vi "Third Flow Restarts Sandbox.vi"() -> ()   [LabVIEW 2013]
uses:
  Type Defs/CAN Mode.ctl
  Type Defs/Controller Names.ctl
  Type Defs/Controller List.ctl
  <vilib>/FPGAPlugInAG/sbRIO-9626/niLvFpga_Open_sbRIO-9626.vi
  <vilib>/rvi/interface/common/dynamic/niFpgaDynamicAddResources.vi
  <vilib>/rvi/interface/common/niFpgaWaitOnOcc.vi
  <vilib>/Utility/error.llb/Error Cluster From Error Code.vi
  <vilib>/rvi/errors/niLvFpgaAdjustHostInterfaceError.vi
  <vilib>/FPGAPlugInAG/Dynamic/niLvFpga_Reset_Dynamic.vi
  <vilib>/FPGAPlugInAG/Dynamic/niLvFpga_Run_Dynamic.vi
  <vilib>/rvi/interface/nirviOpenFPGA/nirviOpenFPGA.xnode
  FPGA/bitfiles/Third Flow Restart Sandbox.lvbitx
  <vilib>/rvi/interface/nirviMethod/nirviMethod.xnode
  <vilib>/rvi/interface/nirviReadWriteControl/nirviReadWriteControl.xnode
  NiFpgaLv.dll
  <vilib>/rvi/interface/Simulation/niFpgaSimulationCallBeginRW.vi
  <vilib>/NI_Real-Time Target Support.lvlib
  <vilib>/FPGAPlugInAG/Dynamic/niLvFpga_ReadFifo_Dynamic.vi
  <vilib>/rvi/errors/niLvFpgaMergeErrorWithErrorCode.vi
  <vilib>/FPGAPlugInAG/Dynamic/niLvFpga_ConfigureFifo_Dynamic.vi
panel:
  out "Cycles":i32
  in  "Reset Cycles":bool
  in  "Continue":bool
  out "Updating?":bool
  out "Starts":i32[](array[numeric])
  in  "Take Trace":bool
  out "tracker":u32
  out "Flow Graphs":dbl[][](graph)
  out "Current Graphs":dbl[][](graph)
  out "Restarts Graph":i32[][](graph)
  in  "Seconds per Step":dbl=1.5 min=0.25 max=500.0 step=0.25
  out "Case":string
  out "Current Step":i32
  in  "Reset Restarts":bool
  in  "Profile":dbl[][](array[numeric])=[[0.25, 0.0, 0.0, 1.0], [1.25, 650.0, 700.0, 0.0], [10.5, 0.0, 0.0, 0.0]]
  in  "Run profile?":bool
  out "CFR 2":u64 format="%.0x"
  in  "Pressure":dbl min=0.0 max=800.0 step=1.0 format="%#_13g"
  out "CPU Usage:":dbl=7.74131899555212 format="%.1f"
  in  "CAN CMD":dbl min=0.0 max=800.0 step=1.0
  # "cmd"
  # "pres"
  # "trigger"
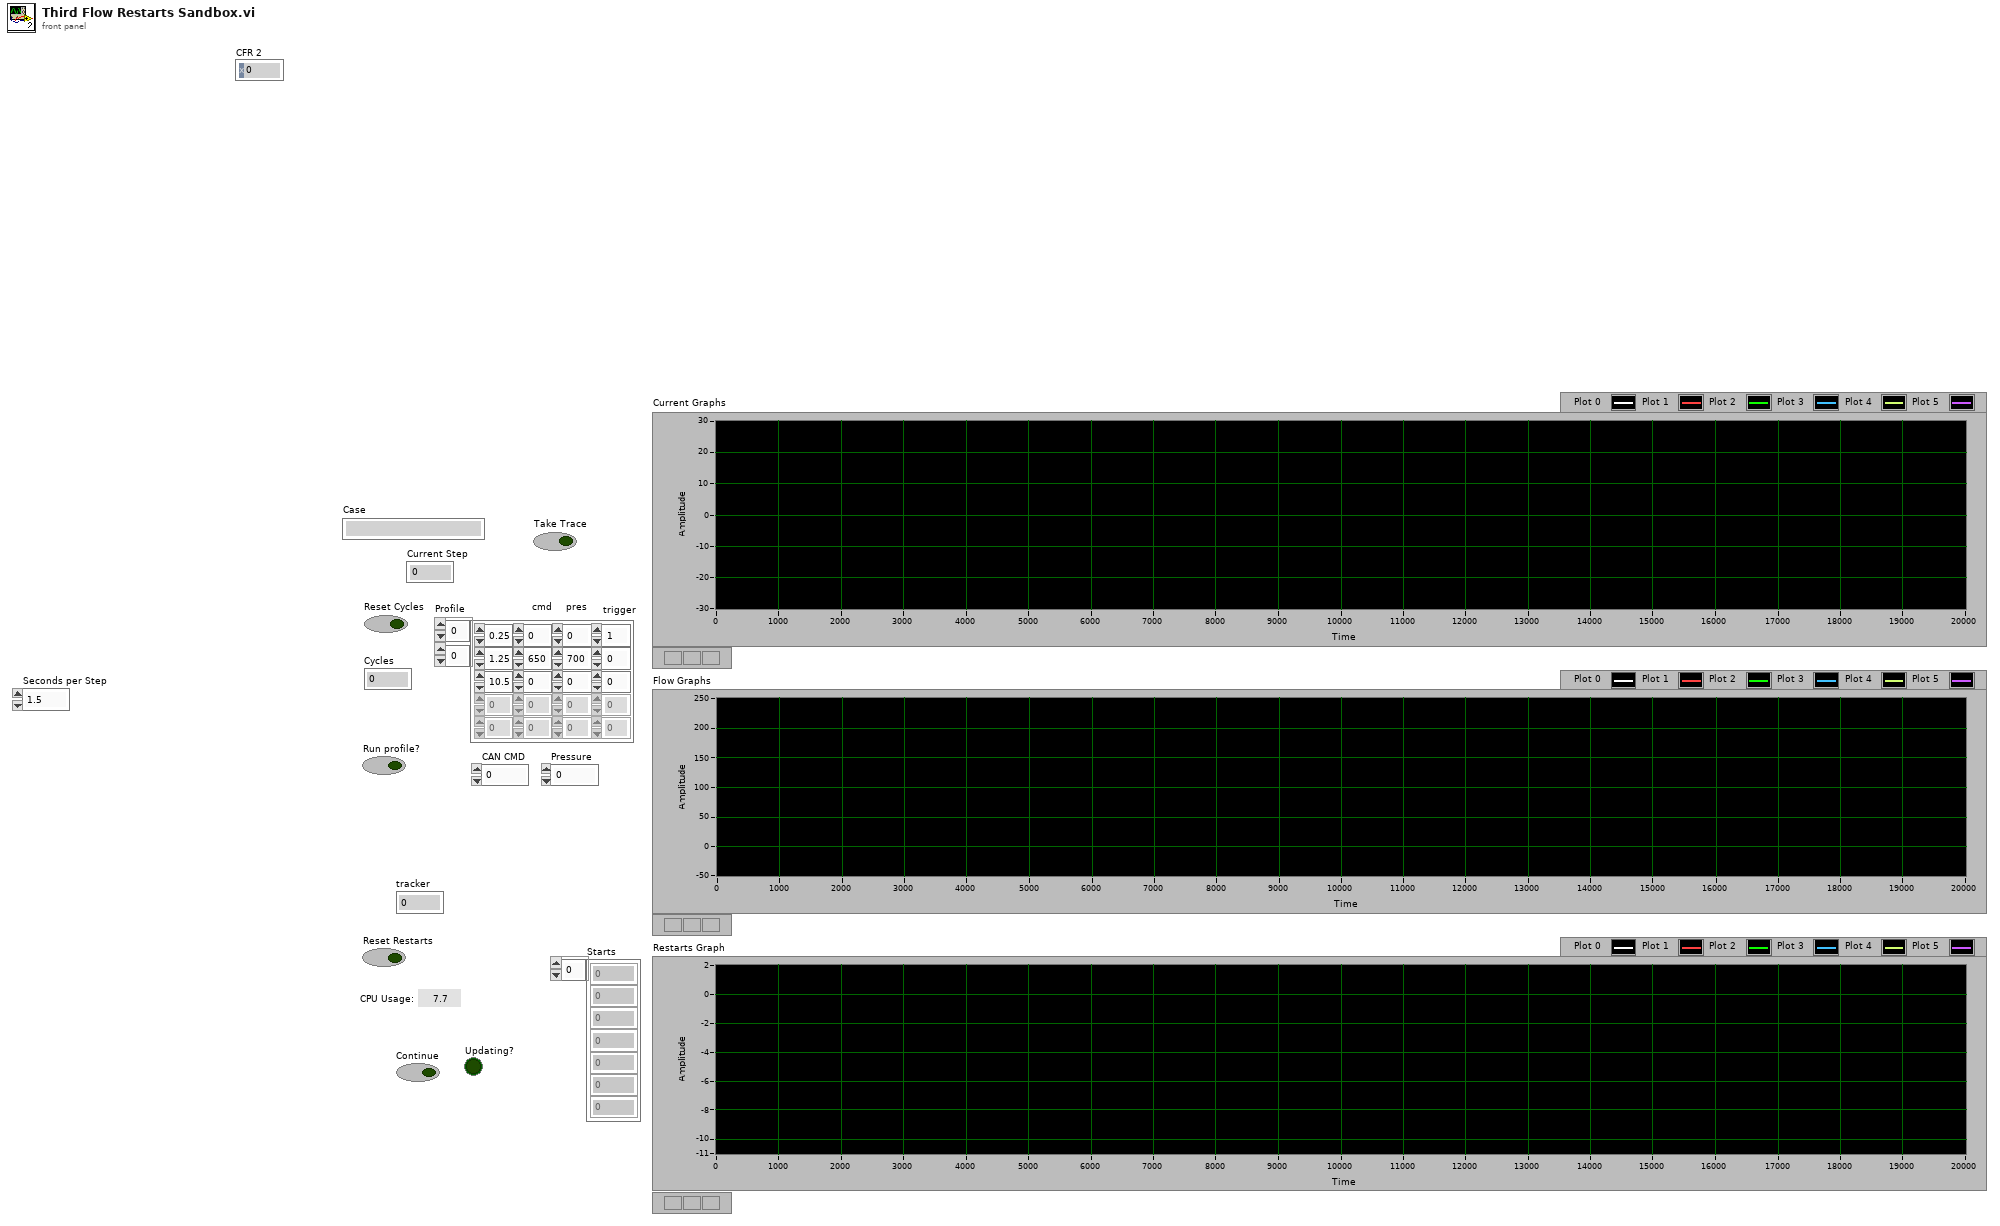
[diagram p1: front panel]
types:
  T1 = typedef "CAN Mode.ctl" = enum16{"Init", "Read", "Write", "Close"}
  T2 = typedef "Controller Names.ctl" = enum16{"Kuhnke", "Conti", "Helbako", "TI PWM", "PSA", "Hella Gas", "Hella Diesel", "8 Comm", "10 Comm", "8 Comm Hella", "10 Comm Hella", "8 Comm Omron", "10 Comm Omron", "8 Comm Nissan", "10 Comm Nissan"}
  T3 = typedef "Controller List.ctl" = cluster{"Controller Name":T2, "CommSeg":i32, "PWM?":bool, "Frequency":i32, "Low Command":dbl, "High Command":dbl, "Stop Command":dbl, "Command Step":dbl, "Solenoid Stop?":bool, "Controller?":bool}[]
  T4 = cluster{"Divide Value":u8, "Transfer Length (bits)":u8, "CS Asserted Polarity":bool, "Clock Polarity (CPOL)":bool, "Clock Phase (CPHA)":bool, "Lengthen MISO Setup":bool, "Direction Change Bit":u8, "MOSI Starts as Output":bool, "Tristatable MOSI":bool}
  T5 = cluster{"Controller Name":T2, "CommSeg":i32, "PWM?":bool, "Frequency":i32, "Low Command":dbl, "High Command":dbl, "Stop Command":dbl, "Command Step":dbl, "Solenoid Stop?":bool, "Controller?":bool}
  T6 = typedef "NI_Real-Time Target Support.lvlib/RT CPU Load.ctl" = cluster{"Total (%)":dbl, "Time Critical (%)":dbl, "Timed Structures (%)":dbl, "High (%)":dbl, "Above Normal (%)":dbl, "Normal (%)":dbl, "Background (%)":dbl, "Idle (%)":dbl, "ISR (%)":dbl}
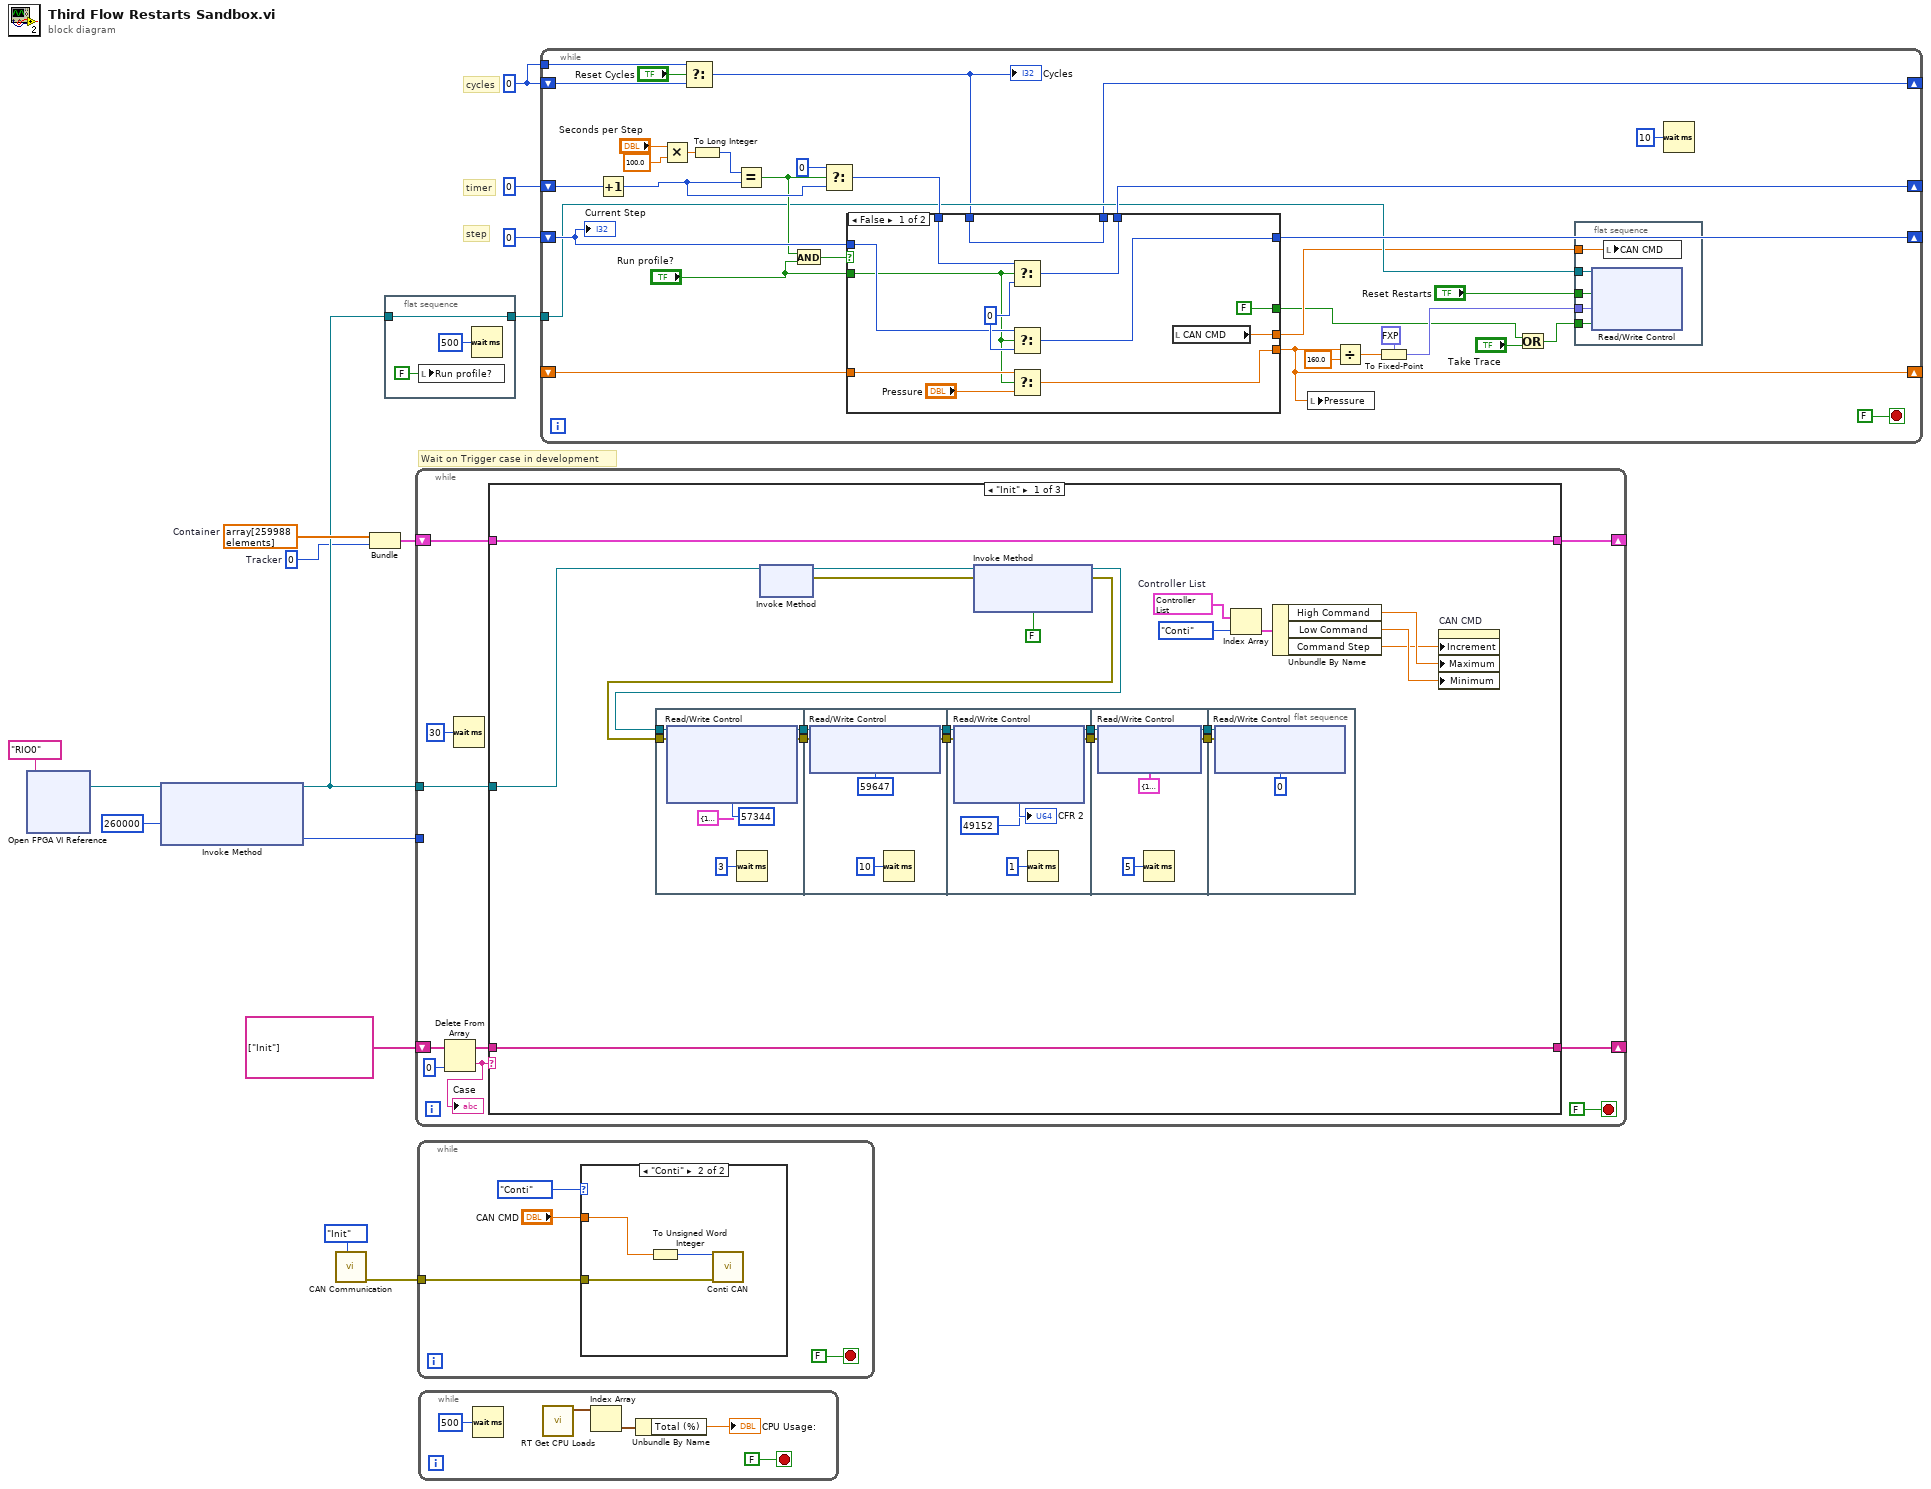
[diagram p0: block diagram]
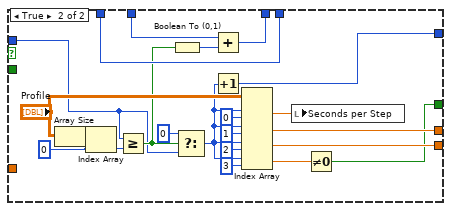
[diagram p2: hidden frame]
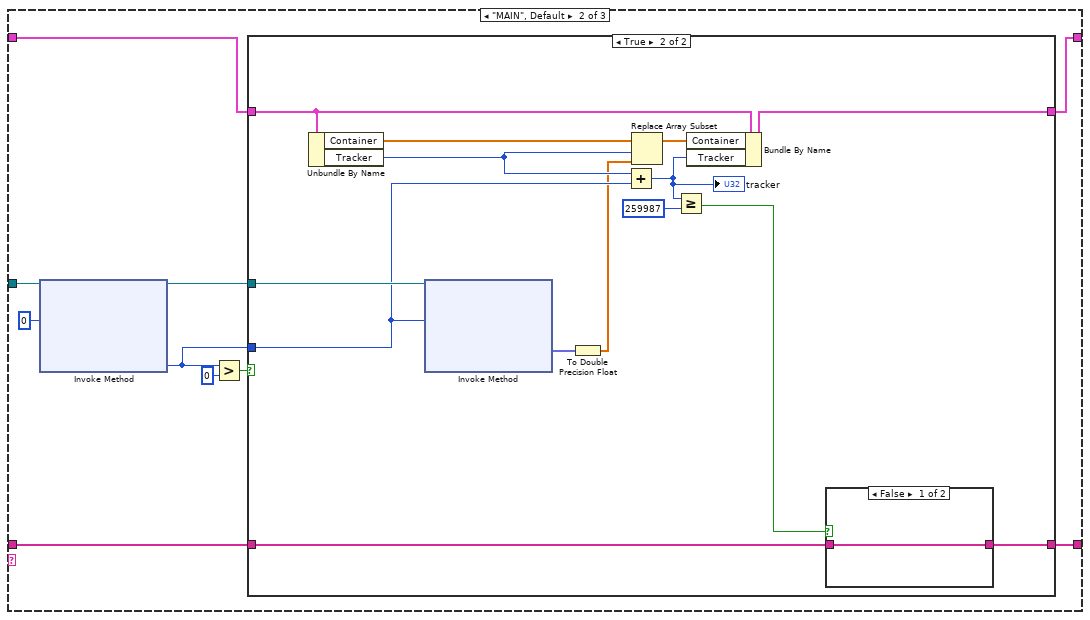
[diagram p3: hidden frame]
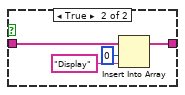
[diagram p5: hidden frame]
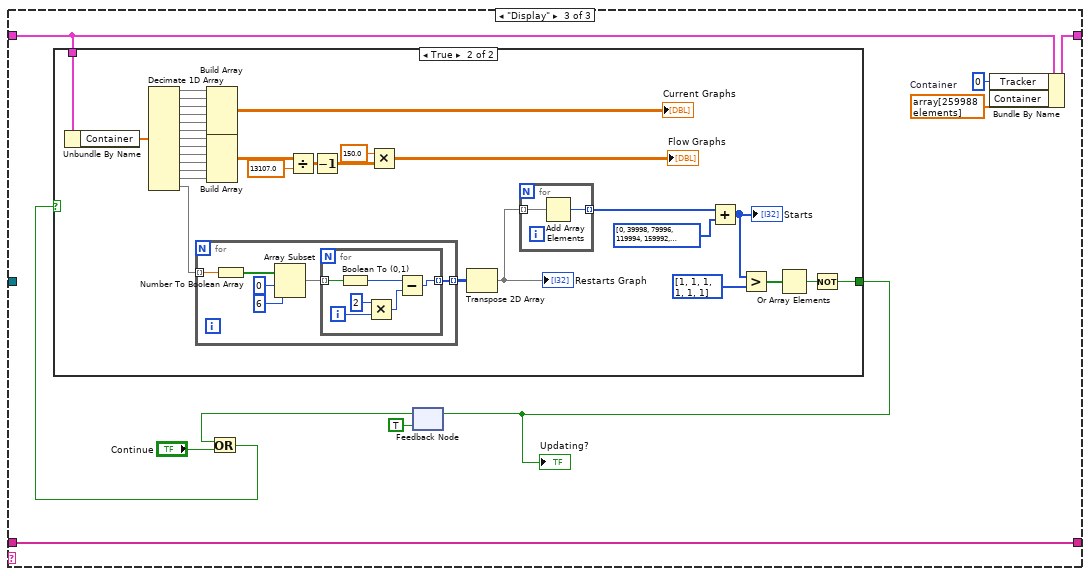
[diagram p6: hidden frame]
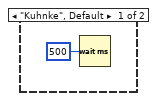
[diagram p8: hidden frame]
diagram:
  w1 = 0 ("disabled index (col)")
  w3 = u32 0  # Tracker
  w7 = dbl[] array[259988 elements]  # Container
  # "cycles"
  # "timer"
  # "step"
  # "Wait on Trigger case in development"
  n1 = xnode "Open FPGA VI Reference"("resource name"=tag "RIO0") -> ("FPGA VI Reference Out"=w9:refnum<k20>)  [unwired: 1 in, 1 out]
  n2 = xnode "Invoke Method"("FPGA VI Reference In"=w9, "Requested Depth"=u32 260000) -> ("FPGA VI Reference Out"=w6:refnum<k20>, "Actual Depth"=w8:u32)  [unwired: 1 in, 1 out]
  n3 = call "CAN Communication.vi"("CAN Mode"=CAN_Mode."Init") -> ("Error OUT"=w13:errorcluster)  [unwired: 10 in]
  n4 = Bundle("Container"=w7, "Tracker"=w3) -> (w11:cluster{"Container":dbl[], "Tracker":u32})  [unwired: 1 in]
  n5 = flat-sequence {
    tunnel: w6 -> [w18]
    tunnel: [w18] -> w2
    frame #0 {
      n6 = local write "Run profile?"(FALSE ("Run profile?")) -> ()
      n7 = Wait (ms)(milliseconds to wait=u32 500) -> ()  [unwired: 1 out]
    }
  }
  n8 = while {
    shift-right: [w25] -> _
    shift-left: string[] ["Init"] -> [w28]
    shift-right: [w22] -> _
    shift-left: w11 -> [w23]
    tunnel: w6 -> [w21]
    tunnel: w8 -> [_]
    stop <- FALSE stop-if-true
    n9 = Delete From Array(array=w28, index=0) -> (deleted portion=w19:string, array with subset deleted=w26:string[])  [unwired: 1 in]
    "Case" <- w19
    n10 = Wait (ms)(milliseconds to wait=u32 30) -> ()  [unwired: 1 out]
    n11 = case shown="\"Init\"" w19 {
      tunnel: w26 -> [w50 w86 w120]
      tunnel: [w50 w85 w120] -> w25
      tunnel: w23 -> [w49 w83 w116]
      tunnel: [w49 w82 w119] -> w22
      tunnel: w21 -> [w48 w89 _]
      frame "Init" {
        w30 = T3 [{"Controller Name"=enum."Kuhnke", "CommSeg"=2, "PWM?"=TRUE, "Frequency"=100, "Low Command"=10.0, "High Command"=100.0, "Stop Command"=10.0, "Command Step"=0.1, "Solenoid Stop?"=FALSE, "Controller?"=FALSE}, {"Controller Name"=enum."Conti", "CommSeg"=2, "PWM?"=FALSE, "Frequency"=100, "Low Command"=0.0, "High Command"=800.0, "Stop Command"=0.0, "Command Step"=1.0, "Solenoid Stop?"=FALSE, "Controller?"=FALSE}, {"Controller Name"=enum."Helbako", "CommSeg"=2, "PWM?"=FALSE, "Frequency"=100, "Low Command"=0.0, "High Command"=100.0, "Stop Command"=0.0, "Command Step"=0.1, "Solenoid Stop?"=FALSE, "Controller?"=FALSE}, {"Controller Name"=enum."TI PWM", "CommSeg"=2, "PWM?"=TRUE, "Frequency"=100, "Low Command"=0.0, "High Command"=100.0, "Stop Command"=0.0, "Command Step"=0.1, "Solenoid Stop?"=FALSE, "Controller?"=FALSE}, {"Controller Name"=enum."PSA", "CommSeg"=2, "PWM?"=TRUE, "Frequency"=100, "Low Command"=5.0, "High Command"=95.0, "Stop Command"=5.0, "Command Step"=0.1, "Solenoid Stop?"=FALSE, "Controller?"=FALSE}, {"Controller Name"=enum."Hella Gas", "CommSeg"=2, "PWM?"=FALSE, "Frequency"=100, "Low Command"=0.0, "High Command"=800.0, "Stop Command"=0.0, "Command Step"=1.0, "Solenoid Stop?"=TRUE, "Controller?"=FALSE}, {"Controller Name"=enum."Hella Diesel", "CommSeg"=2, "PWM?"=FALSE, "Frequency"=100, "Low Command"=370.0, "High Command"=461.0, "Stop Command"=370.0, "Command Step"=1.0, "Solenoid Stop?"=TRUE, "Controller?"=FALSE}, {"Controller Name"=enum."8 Comm", "CommSeg"=8, "PWM?"=FALSE, "Frequency"=100, "Low Command"=0.0, "High Command"=1.0, "Stop Command"=0.0, "Command Step"=1.0, "Solenoid Stop?"=FALSE, "Controller?"=FALSE}, {"Controller Name"=enum."10 Comm", "CommSeg"=10, "PWM?"=FALSE, "Frequency"=100, "Low Command"=0.0, "High Command"=1.0, "Stop Command"=0.0, "Command Step"=1.0, "Solenoid Stop?"=FALSE, "Controller?"=FALSE}, {"Controller Name"=enum."8 Comm Hella", "CommSeg"=8, "PWM?"=TRUE, "Frequency"=150, "Low Command"=0.0, "High Command"=50.0, "Stop Command"=80.0, "Command Step"=0.1, "Solenoid Stop?"=FALSE, "Controller?"=FALSE}, {"Controller Name"=enum."10 Comm Hella", "CommSeg"=10, "PWM?"=TRUE, "Frequency"=150, "Low Command"=0.0, "High Command"=50.0, "Stop Command"=80.0, "Command Step"=0.1, "Solenoid Stop?"=FALSE, "Controller?"=FALSE}, {"Controller Name"=enum."8 Comm Omron", "CommSeg"=8, "PWM?"=TRUE, "Frequency"=150, "Low Command"=5.0, "High Command"=50.0, "Stop Command"=75.0, "Command Step"=0.1, "Solenoid Stop?"=FALSE, "Controller?"=FALSE}, {"Controller Name"=enum."10 Comm Omron", "CommSeg"=10, "PWM?"=TRUE, "Frequency"=150, "Low Command"=5.0, "High Command"=50.0, "Stop Command"=75.0, "Command Step"=0.1, "Solenoid Stop?"=FALSE, "Controller?"=FALSE}, {"Controller Name"=enum."8 Comm Nissan", "CommSeg"=8, "PWM?"=TRUE, "Frequency"=10, "Low Command"=50.0, "High Command"=90.0, "Stop Command"=50.0, "Command Step"=0.1, "Solenoid Stop?"=TRUE, "Controller?"=FALSE}, {"Controller Name"=enum."10 Comm Nissan", "CommSeg"=10, "PWM?"=TRUE, "Frequency"=10, "Low Command"=50.0, "High Command"=90.0, "Stop Command"=50.0, "Command Step"=0.1, "Solenoid Stop?"=TRUE, "Controller?"=FALSE}]  # Controller List
        n12 = flat-sequence {
          tunnel: w34 -> [w56]
          tunnel: w33 -> [w54]
          tunnel: [w57] -> w42
          tunnel: [w55] -> w41
          tunnel: w42 -> [w63]
          tunnel: w41 -> [w62]
          tunnel: [w61] -> w40
          tunnel: [w60] -> w39
          tunnel: w40 -> [w69]
          tunnel: w39 -> [w68]
          tunnel: [w67] -> w38
          tunnel: [w66] -> w37
          tunnel: w38 -> [w76]
          tunnel: w37 -> [w75]
          tunnel: [w73] -> w36
          tunnel: [w72] -> w35
          tunnel: w36 -> [w79]
          tunnel: w35 -> [w78]
          frame #0 {
            w51 = T4 {"Divide Value"=1, "Transfer Length (bits)"=16, "CS Asserted Polarity"=FALSE, "Clock Polarity (CPOL)"=TRUE, "Clock Phase (CPHA)"=FALSE, "Lengthen MISO Setup"=FALSE, "Direction Change Bit"=0, "MOSI Starts as Output"=FALSE, "Tristatable MOSI"=FALSE} ("Master Settings")
            w52 = u64 57344 ("data to write")
            n13 = xnode "Read/Write Control"("FPGA VI Reference In"=w56, "error in"=w54, "AI16-23 Settings"=w51, "AI16-23 Data to Write"=w52, "AI24-31 Settings"=w51, "AI24-31 Data to Write"=w52) -> ("FPGA VI Reference Out"=w57:refnum<k20>, "error out"=w55:errorcluster)
            n14 = Wait (ms)(milliseconds to wait=u32 3) -> ()  [unwired: 1 out]
          }
          frame #1 {
            w58 = u64 59647 ("data to write")
            n15 = xnode "Read/Write Control"("FPGA VI Reference In"=w63, "error in"=w62, "AI16-23 Data to Write"=w58, "AI24-31 Data to Write"=w58) -> ("FPGA VI Reference Out"=w61:refnum<k20>, "error out"=w60:errorcluster)
            n16 = Wait (ms)(milliseconds to wait=u32 10) -> ()  [unwired: 1 out]
          }
          frame #2 {
            w64 = u64 49152 ("data to write")
            n17 = xnode "Read/Write Control"("FPGA VI Reference In"=w69, "error in"=w68, "AI16-23 Data to Write"=w64, "AI24-31 Data to Write"=w64) -> ("FPGA VI Reference Out"=w67:refnum<k20>, "error out"=w66:errorcluster, "Read Data"=→"CFR 2":u64)  [unwired: 1 out]
            n18 = Wait (ms)(milliseconds to wait=u32 1) -> ()  [unwired: 1 out]
          }
          frame #3 {
            w71 = T4 {"Divide Value"=1, "Transfer Length (bits)"=19, "CS Asserted Polarity"=FALSE, "Clock Polarity (CPOL)"=TRUE, "Clock Phase (CPHA)"=FALSE, "Lengthen MISO Setup"=FALSE, "Direction Change Bit"=0, "MOSI Starts as Output"=FALSE, "Tristatable MOSI"=FALSE} ("Master Settings")
            n19 = xnode "Read/Write Control"("FPGA VI Reference In"=w76, "error in"=w75, "AI16-23 Settings"=w71, "AI24-31 Settings"=w71) -> ("FPGA VI Reference Out"=w73:refnum<k20>, "error out"=w72:errorcluster)
            n20 = Wait (ms)(milliseconds to wait=u32 5) -> ()  [unwired: 1 out]
          }
          frame #4 {
            w77 = u64 0 ("AI16-23 Data to Write")
            n21 = xnode "Read/Write Control"("FPGA VI Reference In"=w79, "error in"=w78, "AI16-23 Data to Write"=w77, "AI24-31 Data to Write"=w77) -> ()  [unwired: 2 out]
          }
        }
        n22 = xnode "Invoke Method"("FPGA VI Reference In"=w48) -> ("FPGA VI Reference Out"=w32:refnum<k20>, "error out"=w31:errorcluster)  [unwired: 1 in]
        n23 = xnode "Invoke Method"("FPGA VI Reference In"=w32, "error in"=w31, "Wait Until Done (F)"=FALSE) -> ("FPGA VI Reference Out"=w34:refnum<k20>, "error out"=w33:errorcluster)
        n24 = Index Array(array=w30, index=Controller_Names."Conti" ("Controller Type:")) -> (element=w44:T5)
        n25 = Unbundle By Name(w44) -> ("High Command"=w47:dbl, "Low Command"=w46:dbl, "Command Step"=w45:dbl)
        n26 = property on="CAN CMD" class="DigNum (strict)"("Increment"=w45, "Maximum"=w47, "Minimum"=w46) -> ()  [unwired: 2 in, 2 out]
      }
      frame "MAIN", Default {
        n27 = xnode "Invoke Method"("FPGA VI Reference In"=w89, "Number of Elements"=u32 0) -> ("FPGA VI Reference Out"=w81:refnum<k20>, "Elements Remaining"=w80:u32)  [unwired: 2 in, 2 out]
        n28 = Greater?(x=w80, y=u32 0) -> (0:w84:bool)
        n29 = case shown="True" w84 {
          tunnel: w86 -> [w91 w104]
          tunnel: [w91 w103] -> w85
          tunnel: w83 -> [w90 w100]
          tunnel: [w90 w105] -> w82
          tunnel: w81 -> [_ w101]
          tunnel: w80 -> [_ w99]
          frame False {
          }
          frame True {
            n30 = Unbundle By Name(w100) -> ("Container"=w98:dbl[], "Tracker"=w97:u32)
            n31 = xnode "Invoke Method"("FPGA VI Reference In"=w101, "Number of Elements"=w99) -> ("Data"=w102:fxp<+/-,28,17>[])  [unwired: 2 in, 3 out]
            n32 = To Double Precision Float(number=w102) -> (double precision float=w95:dbl[])
            n33 = Add(x=w97, y=w99) -> (x+y=w94:u32)
            "tracker" <- w94
            n34 = Replace Array Subset(array=w98, new element=w95, index=w97) -> (w96:dbl[])
            n35 = Greater Or Equal?(x=w94, y=u32 259987) -> (x >= y?=w92:bool)
            n36 = Bundle By Name(cluster=w100, "Container"=w96, "Tracker"=w94) -> (w105:cluster{"Container":dbl[], "Tracker":u32})
            n37 = case shown="False" w92 {
              tunnel: w104 -> [w106 w110]
              tunnel: [w106 w109] -> w103
              frame False {
              }
              frame True {
                n38 = Insert Into Array(array=w110, index=0, new element="Display" ("new element/subarray")) -> (w109:string[])
              }
            }
          }
        }
      }
      frame "Display" {
        w117 = dbl[] array[259988 elements]  # Container
        n39 = feedback #1(TRUE) -> (w114:bool)
        n40 = Or(x=w114, y="Continue") -> (x .or. y?=w112:bool)
        n41 = case shown="True" w112 {
          selector: w112 -> [w121 _]
          tunnel: w116 -> [_ w152]
          tunnel: [w121 w122] -> w115
          frame False {
          }
          frame True {
            n42 = Unbundle By Name(w152) -> ("Container"=w151:dbl[])
            n43 = Decimate 1D Array(w151) -> (w150:dbl[], w139:dbl[], w140:dbl[], w141:dbl[], w142:dbl[], w149:dbl[], w148:dbl[], w143:dbl[], w144:dbl[], w145:dbl[], w146:dbl[], w147:dbl[], w131:dbl[])
            n44 = for {
              tunnel: w131 -> [w160] mode=indexing
              tunnel: [w155] -> w130 mode=indexing
              n45 = Number To Boolean Array(number=w160) -> (Boolean array=w159:bool[])
              n46 = Array Subset(array=w159, index=0, length=6) -> (w156:bool[])
              n47 = for {
                tunnel: w156 -> [w166] mode=indexing
                tunnel: [w165] -> w155 mode=indexing
                i -> [w163]
                n48 = Boolean To (0,1)(Boolean=w166) -> (0, 1=w161:i16)
                n49 = Multiply(x=2, y=w163) -> (x*y=w162:i32)
                n50 = Subtract(x=w161, y=w162) -> (x-y=w165:i32)
              }
            }
            n51 = Build Array(w150, w139, w140, w141, w142, w149) -> (→"Current Graphs":dbl[][])
            n52 = Build Array(w148, w143, w144, w145, w146, w147) -> (w138:dbl[][])
            n53 = Divide(x=w138, y=13107.0) -> (x/y=w135:dbl[][])
            n54 = Decrement(x=w135) -> (x-1=w136:dbl[][])
            n55 = Multiply(x=150.0, y=w136) -> (x*y=→"Flow Graphs":dbl[][])
            n56 = Transpose 2D Array(2D array=w130) -> (transposed array=w129:i32[][])
            "Restarts Graph" <- w129
            n57 = for {
              tunnel: w129 -> [w154] mode=indexing
              tunnel: [w153] -> w128 mode=indexing
              n58 = Add Array Elements(numeric array=w154) -> (sum=w153:i32)
            }
            n59 = Add(x=w128, y=i32[] [0, 39998, 79996, 119994, 159992, 199990] ("Starts")) -> (x+y=w126:i32[])
            "Starts" <- w126
            n60 = Greater?(x=w126, y=i32[] [1, 1, 1, 1, 1, 1]) -> (0:w124:bool[])
            n61 = Or Array Elements(Boolean array=w124) -> (logical OR=w123:bool)
            n62 = Not(x=w123) -> (.not. x?=w122:bool)
          }
        }
        "Updating?" <- w115
        n63 = feedback-in #1(w115) -> ()
        n64 = Bundle By Name(cluster=w116, "Tracker"=u32 0, "Container"=w117) -> (w119:cluster{"Container":dbl[], "Tracker":u32})
      }
    }
  }
  n65 = while {
    tunnel: w13 -> [w169]
    stop <- FALSE stop-if-true
    n66 = case shown="\"Conti\"" Controller_Names."Conti" ("Controller Type:") {
      tunnel: w169 -> [_ w174]
      tunnel: "CAN CMD" -> [_ w173]
      frame "Kuhnke", Default {
        n67 = Wait (ms)(milliseconds to wait=u32 500) -> ()  [unwired: 1 out]
      }
      frame "Conti" {
        n68 = To Unsigned Word Integer(number=w173) -> (unsigned 16bit integer=w172:u16)
        n69 = call "Conti CAN.vi"("Error IN"=w174, "CMD"=w172) -> ()  [unwired: 9 in, 1 out]
      }
    }
  }
  n70 = while {
    stop <- FALSE stop-if-true
    n71 = Wait (ms)(milliseconds to wait=u32 500) -> ()  [unwired: 1 out]
    n72 = call <vilib>:"RT Get CPU Loads.vi"() -> ("CPU loads"=w176:T6[])  [unwired: 10 in, 1 out]
    n73 = Index Array(array=w176) -> (element=w177:T6)  [unwired: 1 in]
    n74 = Unbundle By Name(w177) -> ("Total (%)"=→"CPU Usage:":dbl)
  }
  n75 = while {
    tunnel: w2 -> [w195]
    shift-right: [w206] -> _
    shift-left: 0 ("disabled index (col)") -> [w207]
    shift-right: [w201] -> _
    shift-left: 0 ("disabled index (col)") -> [w205]
    shift-right: [w190] -> _
    shift-left: _ -> [w199]
    shift-right: [w181] -> _
    shift-left: w1 -> [w182]
    tunnel: w1 -> [w183]
    stop <- FALSE stop-if-true
    n76 = Increment(x=w205) -> (x+1=w200:i32)
    n77 = Multiply(x="Seconds per Step", y=100.0) -> (x*y=w193:dbl)
    n78 = Select(t=w183, s="Reset Cycles", f=w182) -> (s? t:f=w180:i32)
    "Cycles" <- w180
    n79 = To Long Integer(number=w193) -> (32bit integer=w192:i32)
    n80 = Equal?(x=w192, y=w200) -> (x = y?=w198:bool)
    n81 = And(x=w198, y="Run profile?") -> (x .and. y?=w204:bool)
    n82 = Select(t=0, s=w198, f=w200) -> (s? t:f=w202:i32)
    n83 = case shown="False" w204 {
      tunnel: [w225 w249] -> w190
      tunnel: w207 -> [w223 w230]
      tunnel: [w221 w242] -> w206
      tunnel: w202 -> [w229 w243]
      tunnel: [w228 w243] -> w201
      tunnel: "Run profile?" -> [w222 _]
      tunnel: w199 -> [w227 _]
      tunnel: [w220 w241] -> w191
      tunnel: [FALSE w235] -> w187
      tunnel: w180 -> [w218 w234]
      tunnel: [w218 w233] -> w181
      frame False {
        w224 = 0 ("disabled index (col)")
        n84 = Select(t=w229, s=w222, f=w224) -> (s? t:f=w228:i32)
        n85 = Select(t=w223, s=w222, f=w224) -> (s? t:f=w221:i32)
        n86 = Select(t=w227, s=w222, f="Pressure") -> (s? t:f=w225:dbl)
        n87 = local read "CAN CMD"() -> (w220:dbl)
      }
      frame True {
        n88 = Array Size(array="Profile") -> (size(s)=w247:i32[])
        n89 = Index Array(array=w247, index=0 ("disabled index (col)")) -> (element=w245:i32)
        n90 = Greater Or Equal?(x=w230, y=w245) -> (x >= y?=w231:bool)
        n91 = Boolean To (0,1)(Boolean=w231) -> (0, 1=w232:i16)
        n92 = Select(t=0, s=w231, f=w230) -> (s? t:f=w238:i32)
        n93 = Add(x=w234, y=w232) -> (x+y=w233:i32)
        n94 = Increment(x=w238) -> (x+1=w242:i32)
        n95 = Index Array(array="Profile", index (row) #1=w238, index (col) #1=0 ("disabled index (col)"), index (row) #2=w238, index (col) #2=1 ("disabled index (col)"), index (row) #3=w238, index (col) #3=2 ("disabled index (col)"), index (row) #4=w238, index (col) #4=3 ("disabled index (col)")) -> (element #1=w239:dbl, element #2=w241:dbl, element #3=w249:dbl, element #4=w236:dbl)
        n96 = local write "Seconds per Step"(w239) -> ()
        n97 = Not Equal To 0?(x=w236) -> (x != 0?=w235:bool)
      }
    }
    n98 = local write "Pressure"(w190) -> ()
    n99 = Divide(x=w190, y=160.0) -> (x/y=w209:dbl)
    n100 = To Fixed-Point(fixed-point type=fxp<+/-,20,5> 0.0 ("AO0"), number=w209) -> (fixed-point=w208:fxp<+/-,20,5>)
    n101 = Or(x=w187, y="Take Trace") -> (x .or. y?=w186:bool)
    n102 = flat-sequence {
      tunnel: w208 -> [w217]
      tunnel: w195 -> [w216]
      tunnel: "Reset Restarts" -> [w215]
      tunnel: w191 -> [w214]
      tunnel: w186 -> [w213]
      frame #0 {
        n103 = xnode "Read/Write Control"("FPGA VI Reference In"=w216, "Reset Restarts"=w215, "AO0"=w217, "Trigger"=w213) -> ()  [unwired: 1 in, 2 out]
        n104 = local write "CAN CMD"(w214) -> ()
      }
    }
    n105 = Wait (ms)(milliseconds to wait=u32 10) -> ()  [unwired: 1 out]
    "Current Step" <- w207
  }
